vi "support - acquire data.vi"(8 "error in (no error)":errorcluster) -> (0 "error out":errorcluster, 3 "sin(x)":dbl)   [LabVIEW 2015]
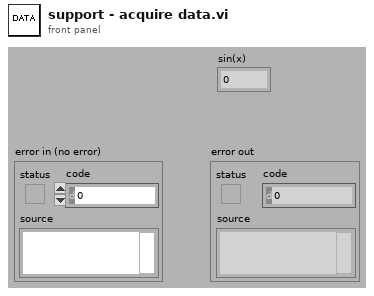
[diagram p1: front panel]
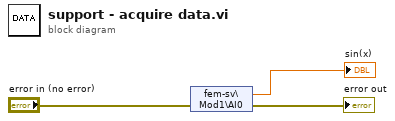
[diagram p0: block diagram]
diagram:
  n1 = shared-variable "fem-sv\\Mod1\\AI0"(error in="error in (no error)") -> (→"sin(x)":dbl, error out=→"error out":errorcluster)
